vi "Export_map2Text.vi"(1 "MapData (2D)":dbl[][](array[numeric]), 2 "XY Full":cluster{dbl, dbl}[](array[cluster]), 3 "ExportPath":path) -> ()   [LabVIEW 2010]
uses:
  <vilib>/Analysis/polynomials.llb/Unique Numbers and Multiplicity (DBL).vi
  <vilib>/Utility/file.llb/Write To Spreadsheet File (DBL).vi
  <vilib>/Analysis/NI_AALPro.lvlib
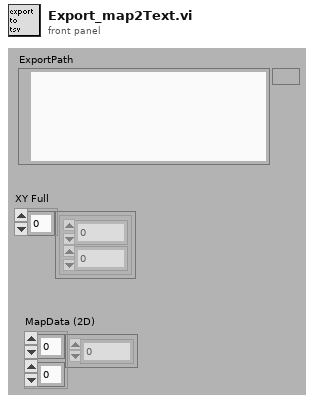
[diagram p1: front panel]
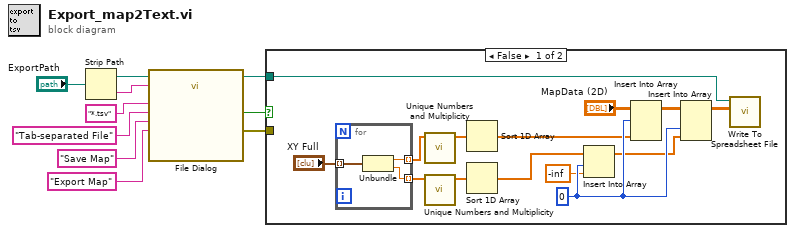
[diagram p0: block diagram]
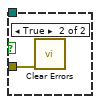
[diagram p2: hidden frame]
diagram:
  n1 = Strip Path(path="ExportPath") -> (stripped path=w6:path, name=w5:string)
  n2 = call "File Dialog"("start path"=w6, "prompt"="Export Map" ("button label"), "button label"="Save Map" ("prompt"), "default name"=w5, "pattern (all files)"="*.tsv", "pattern label"="Tab-separated File") -> ("selected path"=w10:path, "cancelled"=w9:bool, "error out"=w8:errorcluster)  [unwired: 6 in, 1 out]
  n3 = case shown="False" w9 {
    tunnel: w10 -> [w24 _]
    tunnel: w8 -> [_ w28]
    frame False {
      w20 = 0 ("Deaktivierter Index (Spalte)")
      n4 = for {
        tunnel: "XY Full" -> [w27] mode=indexing
        tunnel: [w26] -> w14 mode=indexing
        tunnel: [w25] -> w16 mode=indexing
        n5 = Unbundle(w27) -> (w26:dbl, w25:dbl)
      }
      n6 = call-poly <vilib>:"Unique Numbers and Multiplicity.vi"("Numbers"=w14) -> ("Unique Numbers"=w15:dbl[])  [unwired: 8 in, 2 out]
      n7 = call-poly <vilib>:"Unique Numbers and Multiplicity.vi"("Numbers"=w16) -> ("Unique Numbers"=w17:dbl[])  [unwired: 8 in, 2 out]
      n8 = Sort 1D Array(array=w15) -> (sorted array=w12:dbl[])
      n9 = Sort 1D Array(array=w17) -> (sorted array=w11:dbl[])
      n10 = Insert Into Array(array=w11, index=w20, new element=-inf ("Neues Element/Teil-Array")) -> (w18:dbl[])
      n11 = Insert Into Array(array="MapData (2D)", index (row)=w20, new element=w12) -> (w22:dbl[][])  [unwired: 1 in]
      n12 = Insert Into Array(array=w22, index (col)=w20, new element=w18) -> (w21:dbl[][])  [unwired: 1 in]
      n13 = call-poly <vilib>:"Write To Spreadsheet File.vi"("2D data"=w21, "file path (dialog if empty)"=w24) -> ()  [unwired: 6 in, 1 out]
    }
    frame True {
      n14 = call <vilib>:"Clear Errors.vi"("error in (no error)"=w28) -> ()  [unwired: 6 in, 1 out]
    }
  }
